vi "TimingTestBox_Asynchronous.vi"(0 "Left(100)":i16=100, 5 "Top(100)":i16=100, 7 "定时参数(1000ms)":u32[](array[numeric]), 11 "YT System Queue":refnum<queue>) -> ()   [LabVIEW 2017]
uses:
  YtCommon.lvlibp/yt`Step System Queue.ctl
  <vilib>/Utility/miscctls.llb/LVPointTypeDef.ctl
  <vilib>/Utility/miscctls.llb/LVRectTypeDef.ctl
  YtCommon.lvlibp
panel:
  in  "AutoTestDUTALL":bool caption="全部"
  in  "AutoTestDUT16":bool caption="DUT16"
  in  "AutoTestDUT15":bool caption="DUT15"
  in  "AutoTestDUT14":bool caption="DUT14"
  in  "AutoTestDUT13":bool caption="DUT13"
  in  "AutoTestDUT12":bool caption="DUT12"
  in  "AutoTestDUT11":bool caption="DUT11"
  in  "AutoTestDUT10":bool caption="DUT10"
  in  "AutoTestDUT9":bool caption="DUT9"
  in  "AutoTestDUT8":bool caption="DUT8"
  in  "AutoTestDUT7":bool caption="DUT7"
  in  "AutoTestDUT6":bool caption="DUT6"
  in  "AutoTestDUT5":bool caption="DUT5"
  in  "AutoTestDUT4":bool caption="DUT4"
  in  "AutoTestDUT3":bool caption="DUT3"
  in  "AutoTestDUT2":bool caption="DUT2"
  in  "AutoTestDUT1":bool caption="DUT1"
  in  "logo Button":bool
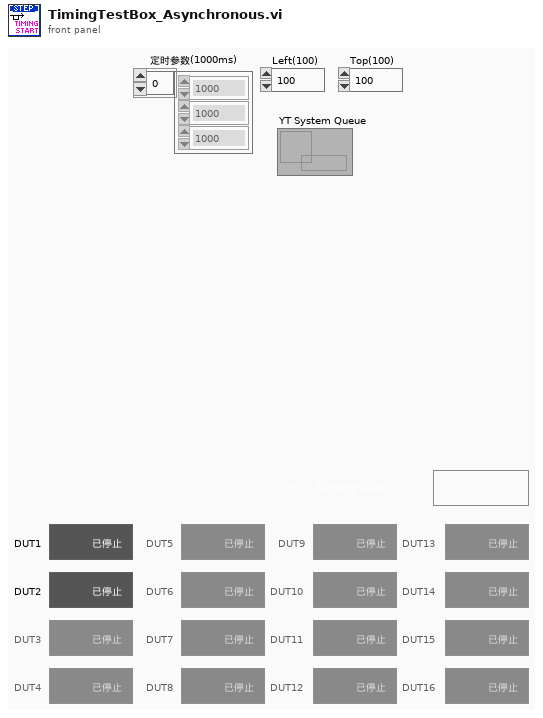
[diagram p1: front panel]
types:
  T1 = typedef "LVRectTypeDef.ctl" = cluster{"Left":i16, "Top":i16, "Right":i16, "Bottom":i16}
  T2 = typedef "LVPointTypeDef.ctl" = cluster{"Horizontal":i16, "Vertical":i16}
  T3 = enum8{"Enabled", "Disabled", "Disabled and Grayed Out"}
  T4 = typedef "YtCommon.lvlibp/yt`Step System Queue.ctl" = cluster{"Socket(From0)":i32, "Cmd":string, "Data":variant}
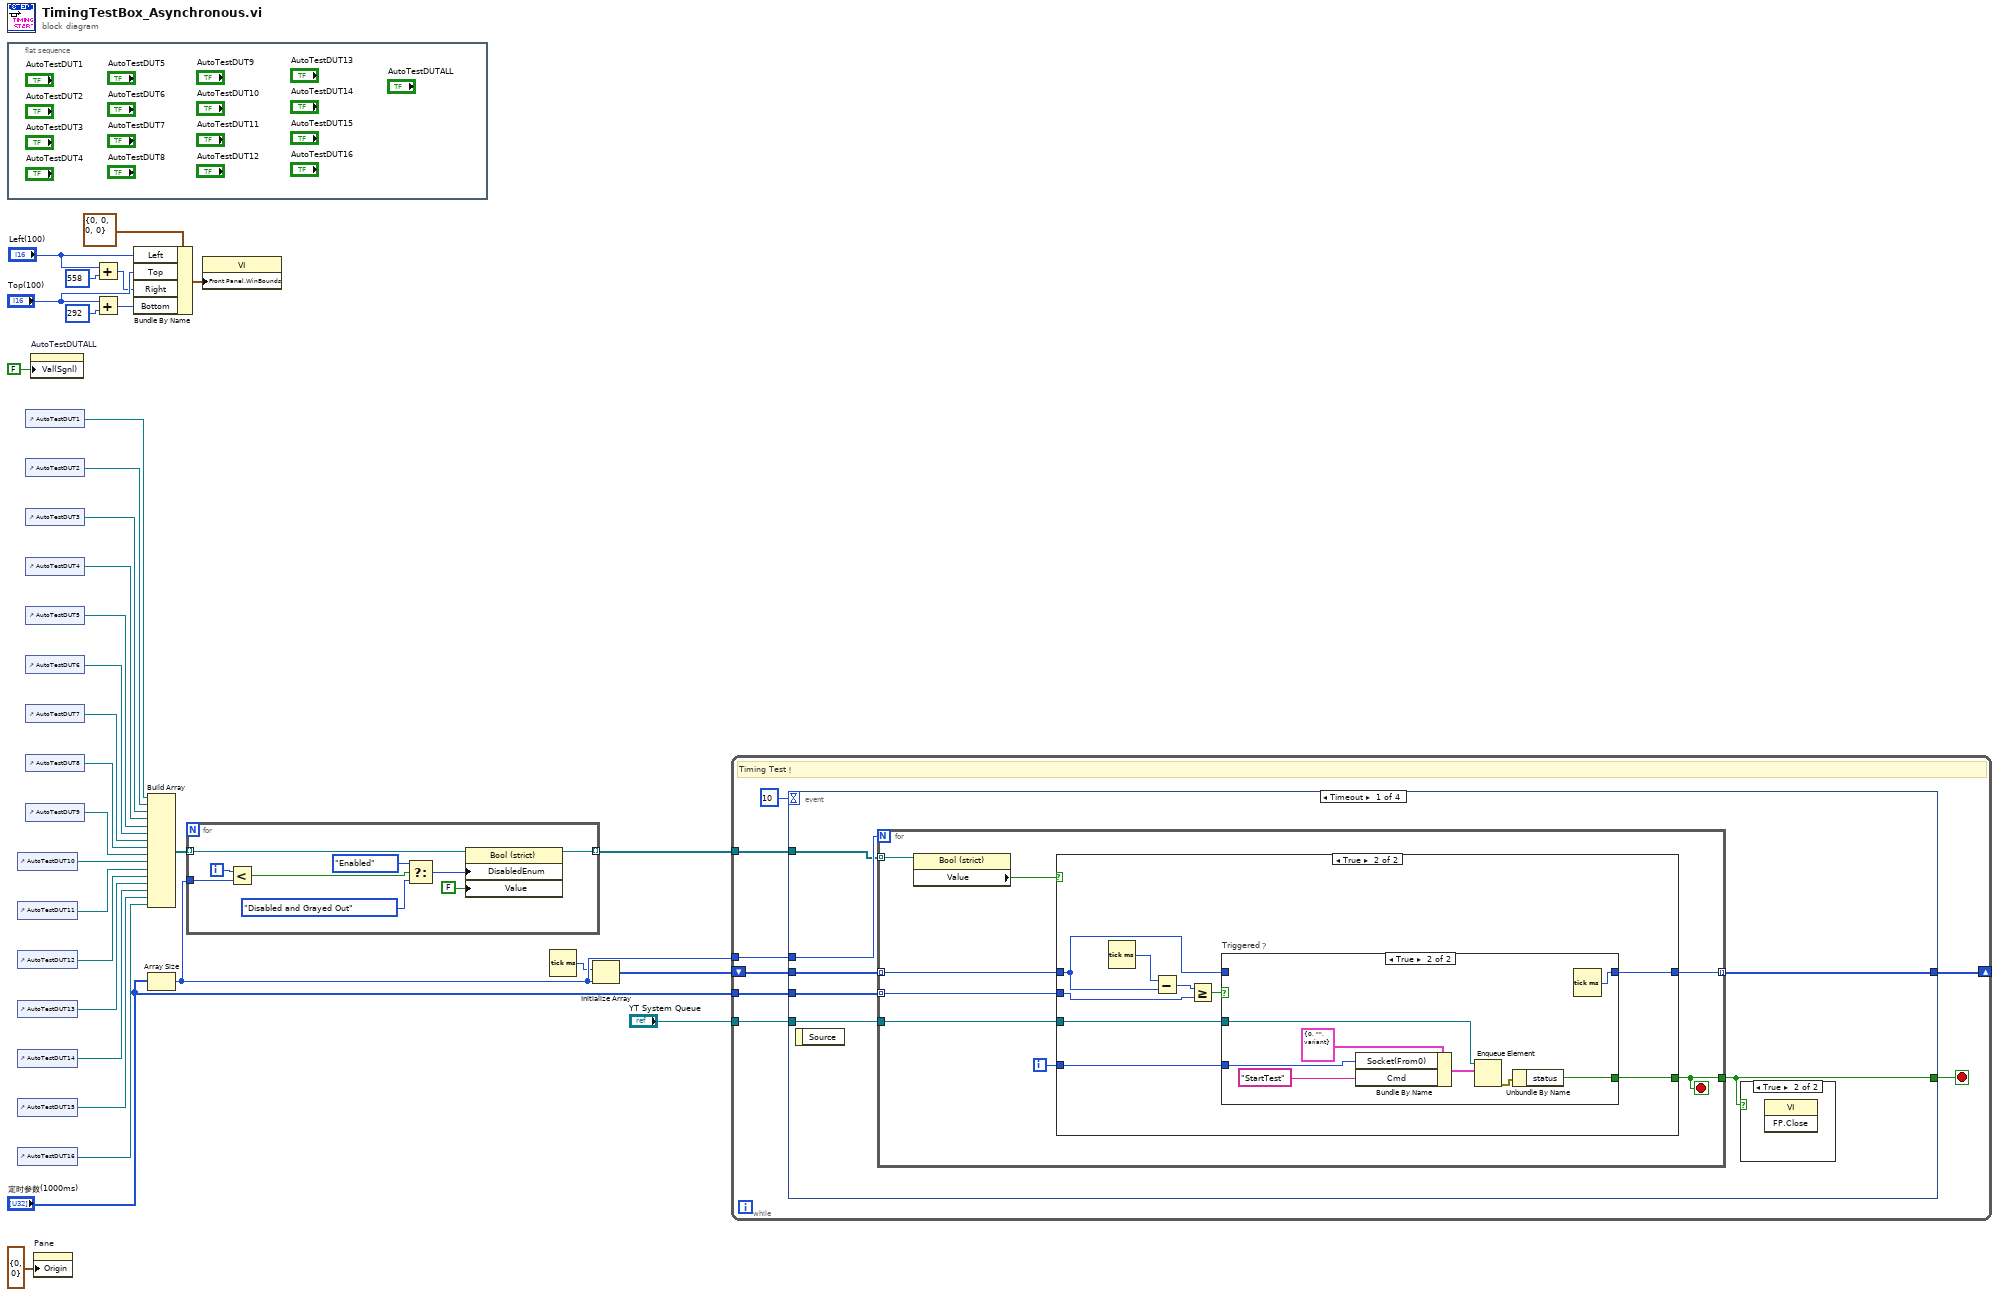
[diagram p0: block diagram]
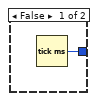
[diagram p3: hidden frame]
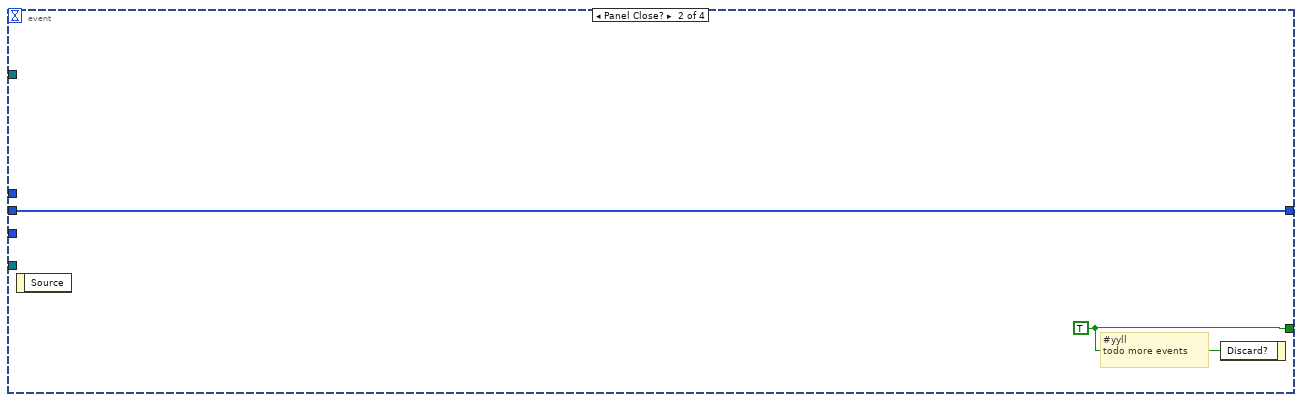
[diagram p5: hidden frame]
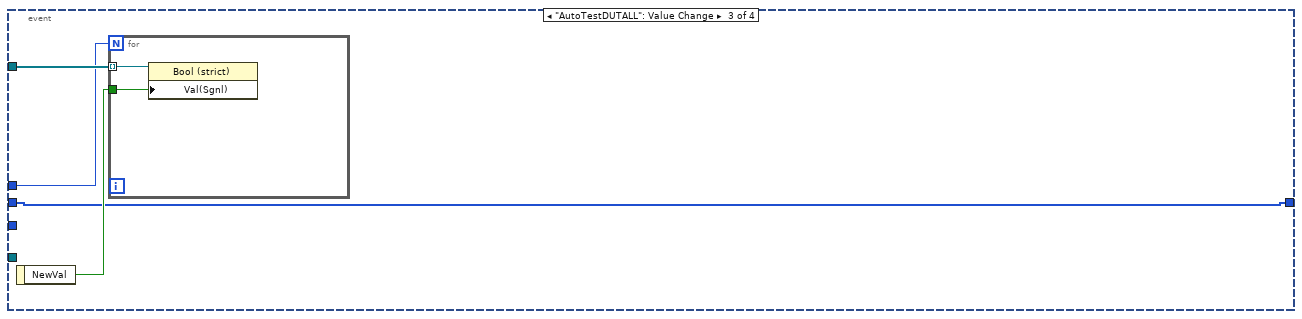
[diagram p6: hidden frame]
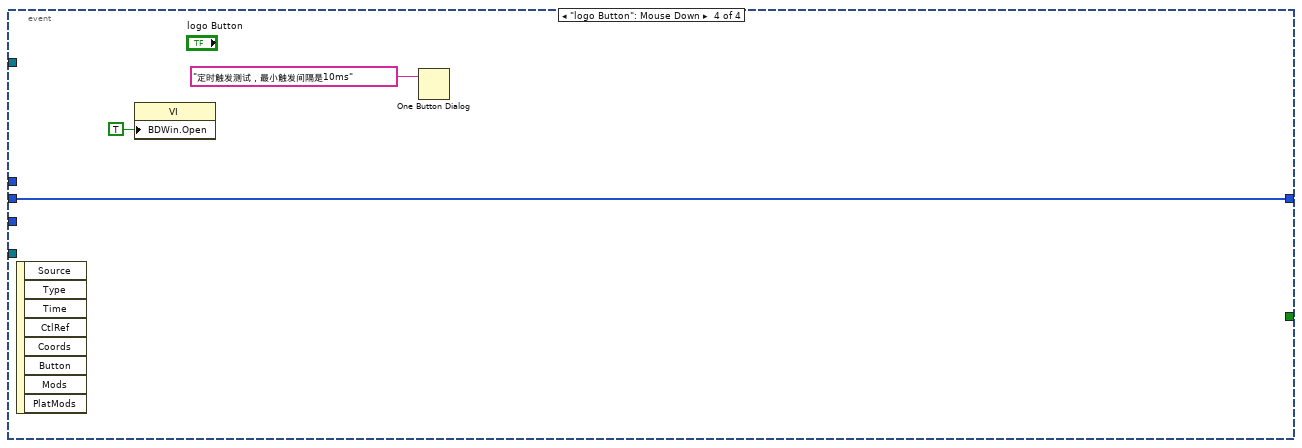
[diagram p7: hidden frame]
diagram:
  n1 = flat-sequence {
    frame #0 {
    }
  }
  n2 = control-ref of="AutoTestDUT10"() -> (w23:refnum<vi>)
  n3 = control-ref of="AutoTestDUT11"() -> (w22:refnum<vi>)
  n4 = control-ref of="AutoTestDUT12"() -> (w21:refnum<vi>)
  n5 = control-ref of="AutoTestDUT13"() -> (w20:refnum<vi>)
  n6 = control-ref of="AutoTestDUT14"() -> (w19:refnum<vi>)
  n7 = control-ref of="AutoTestDUT15"() -> (w18:refnum<vi>)
  n8 = control-ref of="AutoTestDUT16"() -> (w17:refnum<vi>)
  n9 = control-ref of="AutoTestDUT1"() -> (w32:refnum<vi>)
  n10 = control-ref of="AutoTestDUT2"() -> (w31:refnum<vi>)
  n11 = control-ref of="AutoTestDUT3"() -> (w30:refnum<vi>)
  n12 = control-ref of="AutoTestDUT4"() -> (w29:refnum<vi>)
  n13 = control-ref of="AutoTestDUT5"() -> (w28:refnum<vi>)
  n14 = control-ref of="AutoTestDUT6"() -> (w27:refnum<vi>)
  n15 = control-ref of="AutoTestDUT7"() -> (w26:refnum<vi>)
  n16 = control-ref of="AutoTestDUT8"() -> (w25:refnum<vi>)
  n17 = control-ref of="AutoTestDUT9"() -> (w24:refnum<vi>)
  n18 = property on="AutoTestDUTALL" class="Bool (strict)"("Val(Sgnl)"=FALSE ("AutoTestDUTALL")) -> ()  [unwired: 2 in, 2 out]
  n19 = property on="Pane" class="Pane"("Origin"=T2 {"Horizontal"=0, "Vertical"=0}) -> ()  [unwired: 2 in, 2 out]
  n20 = Add(x="Left(100)", y=i16 558) -> (x+y=w13:i16)
  n21 = Add(x="Top(100)", y=i16 292) -> (x+y=w15:i16)
  n22 = Bundle By Name(cluster=T1 {"Left"=0, "Top"=0, "Right"=0, "Bottom"=0} ("Front Panel Window:Window Bounds"), "Left"="Left(100)", "Top"="Top(100)", "Right"=w13, "Bottom"=w15) -> (w11:T1)
  n23 = Build Array(w32, w31, w30, w29, w28, w27, w26, w25, w24, w23, w22, w21, w20, w19, w18, w17) -> (w7:refnum<vi>[])
  n24 = Array Size(array="定时参数(1000ms)") -> (size(s)=w5:i32)
  n25 = for {
    tunnel: w7 -> [w42] mode=indexing
    tunnel: [w41] -> w6 mode=indexing
    tunnel: w5 -> [w39]
    i -> [w40]
    n26 = Less?(x=w40, y=w39) -> (x < y?=w38:bool)
    n27 = Select(t=T3."Enabled" ("Disabled"), s=w38, f=T3."Disabled and Grayed Out" ("Disabled")) -> (s? t:f=w35:T3)
    n28 = property on="Property Node" class="Bool (strict)"(reference=w42, "DisabledEnum"=w35, "Value"=FALSE) -> (reference out=w41:refnum<vi>)  [unwired: 1 in, 1 out]
  }
  n29 = property class="VI"("Front Panel.WinBounds"=w11) -> ()  [unwired: 2 in, 2 out]
  n30 = Tick Count (ms)() -> (millisecond timer value=w4:u32)
  n31 = Initialize Array(w4, w5) -> (w3:u32[])
  n32 = while {
    tunnel: w6 -> [w48]
    tunnel: w5 -> [w47]
    shift-right: [w45] -> _
    shift-left: w3 -> [w46]
    tunnel: "定时参数(1000ms)" -> [w44]
    tunnel: "YT System Queue" -> [w43]
    stop <- w49 stop-if-true
    # "Timing Test！"
    n33 = event shown="[0] Timeout" {
      selector: _ -> [_ _ _ _]
      dyn-events: _ -> [_ _ _ _]
      timeout: 10 -> [_ _ _ _]
      tunnel: [w51 w86 _ _] -> w49
      tunnel: w48 -> [w55 _ w90 _]
      tunnel: w47 -> [w56 _ w88 _]
      tunnel: w46 -> [w57 w85 w87 w93]
      tunnel: [w54 w85 w87 w93] -> w45
      tunnel: w44 -> [w53 _ _ _]
      tunnel: w43 -> [w52 _ _ _]
      event Timeout {
        n34 = event-data() -> ()  [unwired: 1 in, 1 out]
        n35 = for {
          N: w56 -> [_]
          tunnel: w57 -> [w62] mode=indexing
          tunnel: w55 -> [w65] mode=indexing
          tunnel: [w63] -> w54 mode=indexing
          tunnel: w53 -> [w61] mode=indexing
          tunnel: w52 -> [w60]
          tunnel: [w59] -> w51
          i -> [w58]
          stop <- w59 stop-if-true
          n36 = property on="Property Node" class="Bool (strict)"(reference=w65) -> ("Value"=w64:bool)  [unwired: 1 in, 2 out]
          n37 = case shown="True" w64 {
            tunnel: [w66 w71] -> w63
            tunnel: w62 -> [_ w70]
            tunnel: w61 -> [_ w73]
            tunnel: w60 -> [_ w69]
            tunnel: [_ w68] -> w59
            tunnel: w58 -> [_ w67]
            frame False {
              n38 = Tick Count (ms)() -> (millisecond timer value=w66:u32)
            }
            frame True {
              n39 = Tick Count (ms)() -> (millisecond timer value=w75:u32)
              n40 = Subtract(x=w75, y=w70) -> (x-y=w74:u32)
              n41 = Greater Or Equal?(x=w74, y=w73) -> (x >= y?=w72:bool)
              n42 = case "Triggered？" shown="True" w72 {
                tunnel: [w76 w84] -> w71
                tunnel: w70 -> [w76 _]
                tunnel: w69 -> [_ w83]
                tunnel: [_ w81] -> w68
                tunnel: w67 -> [_ w78]
                frame False {
                }
                frame True {
                  n43 = Bundle By Name(cluster=T4 {"Socket(From0)"=0, "Cmd"="", "Data"=variant} ("element"), "Socket(From0)"=w78, "Cmd"="StartTest") -> (w79:T4)
                  n44 = Enqueue Element(queue=w83, element=w79) -> (error out=w82:errorcluster)  [unwired: 2 in, 2 out]
                  n45 = Unbundle By Name(w82) -> ("status"=w81:bool)
                  n46 = Tick Count (ms)() -> (millisecond timer value=w84:u32)
                }
              }
            }
          }
        }
        n47 = case shown="True" w51 {
          frame False {
          }
          frame True {
            n48 = invoke class="VI" method="FP.Close"() -> ()  [unwired: 3 in, 3 out]
          }
        }
      }
      event Panel Close? {
        w86 = TRUE ("Discard?")
        # "#yyll\ntodo more events"
        n49 = event-data() -> ()  [unwired: 1 in, 1 out]
        n50 = event-data("Discard?"=w86) -> ()  [unwired: 1 in, 1 out]
      }
      event "AutoTestDUTALL": Value Change {
        n51 = event-data() -> ("NewVal"=w89:bool)  [unwired: 1 in]
        n52 = for {
          N: w88 -> [_]
          tunnel: w90 -> [w92] mode=indexing
          tunnel: w89 -> [w91]
          n53 = property on="Property Node" class="Bool (strict)"(reference=w92, "Val(Sgnl)"=w91) -> ()  [unwired: 1 in, 2 out]
        }
      }
      event "logo Button": Mouse Down {
        n54 = event-data() -> ()  [unwired: 1 in, 8 out]
        n55 = property class="VI"("BDWin.Open"=TRUE ("Block Diagram Window:Open")) -> ()  [unwired: 2 in, 2 out]
        n56 = One Button Dialog(message="定时触发测试，最小触发间隔是10ms") -> ()  [unwired: 1 in, 1 out]
      }
    }
  }
